vi "Write Image Header.vi"(8 "error in (no error)":errorcluster, 10 "Header Contents":T1={"FILENAME"=["FILENAME", "example.fits", "File name at acquisition"], "OBSERVER"=["OBSERVER", "Denis", "Observer’s (PI) name"], "PROGRID"=["PROGRID", "2018A-001", "Program ID"], "OBJECT"=["OBJECT", "UNDEFINED", "Object name"], "NIGHTDIR"=["NIGHTDIR", "DIR", "Night directory name "], "CHANNEL"=["CHANNEL", "RED", "Instrument channel"], "INSTRUME"=["INSTRUME", "ECHARPE", "Instrument"], "NEXPSEQ"=["NEXPSEQ", "1", "Total number of exposures in sequence"], "SEQINDEX"=["SEQINDEX", "1", "Exposure index in the sequence"], "OBSTYPE"=["OBSTYPE", "BIAS", "Image type: OBJECT, BIAS, FLAT, ARC, DARK"], "READMOD"=["READMOD", "Normal", "Read out mode: fast, normal, slow"], "SHUTTER"=["SHUTTER", "CLOSED", "Shutter Mode (OPEN, CLOSED, or AUTO) "], "OPENSHT"=["OPENSHT", "50", "Time to open the shutter (ms) "], "CLOSESHT"=["CLOSESHT", "50", "Time to close the shutter (ms)"], "GAIN"=["GAIN", "3.38", "Gain (e-/ADU)"], "GAINERR "=["GAINERR", "0.05", " Gain error (e-/ADU)"], "RDNOISE"=["RDNOISE", "6.55", "Read noise (e-)"], "RNOISERR"=["RNOISERR", "0.02", "Read noise error (e-)"], "SKYFIBER"=["SKYFIBER", "\"OFF\"", "Sky fiber: ON or OFF"], "CALFIBER"=["CALFIBER", "\"OFF\"", "Calibration Fiber: ON or OFF"], "UTDATE"=["UTDATE", "'2017-10-01T20", "UT date at start of exposure"], "LOCTIME"=["LOCTIME", "'2017-10-01T17", "LT date at start of exposure"], "MJD"=["MJD", "58027.500000", "Modified Julian Date at start of exposure"], "OBSLON"=["OBSLON", "-45.57972", "Observatory East Longitude"], "OBSLAT"=["OBSLAT", "-22.53444", "Observatory Latitude"], "OBSALT"=["OBSALT", "1864.0", "Observatory elevation above sea level (m)"], "EXPTIME"=["EXPTIME", "1", "Exposure time (s)"], "TELRA"=["TELRA", "“00:00:00.000”", "TCS right ascension: “HH:MM:SS.SSS”"], "TELDEC"=["TELDEC", "“+00:00:00.000”", "TCS declination: “+-DD:MM:SS.SSS”"], "RA"=["RA", "“00:00:00.000”", "Requested right Ascension: “HH:MM:SS.SSS”"], "DEC"=["DEC", "“+00:00:00.000”", "Requested Declination: “+- DD:MM:SS.SSS”"], "RA_DEG"=["RA_DEG", "128.84946", "Requested Right Ascension (deg)"], "DEC_DEG"=["DEC_DEG", "+19.648717", "Requested Declination (deg)"], "EPOCH"=["EPOCH", "2000.00", "Epoch for Target coordinates"], "HA"=["HA", "“+01:13:05.98”", "Hour Angle (Sexagesimal)"], "HAD"=["HAD", "1.2183292", "Hour Angle (deg)"], "AIRMASS"=["AIRMASS", "1.085", "Mean airmass for the observation"], "AMSTART"=["AMSTART", "1.060", "Airmass at start of exposure"], "AMEND"=["AMEND", "1.114", "Airmass at end of exposure"], "XOFFSET"=["XOFFSET", "0.000000", "Telescope RA offset in arcsec"], "YOFFSET"=["YOFFSET", "0.000000", "Telescope DEC offset in arcsec"], "PA"=["PA", "14.6415392418", "Current Rotator Position Angle (degree)"], "CAMFOC"=["CAMFOC", "-3.53", "Camera focus position (mm)"], "TELFOC"=["TELFOC", "-3.53", "Telescope focus position (mm)"], "TCSUT"=["TCSUT", "‘23:17:24.8’", "TCS Universal Time"], "MOONDIST"=["MOONDIST", "60.0", "Moon angular distance to object (deg)"], "MOONALT"=["MOONALT", "15.0", "Moon elevation above horizon (deg)"], "MONNPHAS"=["MOONPHAS", "30.0", "Moon phase (deg)"], "ADC"=["ADC", "\"ON\"", "Atmospheric Dispersion Corrector: ON or OFF"], "ADCSPPED"=["ADCSPPED", "5.0", "ADC motor speed (rpm)"], "CALMIRR"=["CALMIRR", "\"OUT\"", "Calibration mirror position: IN or OUT"], "GUIDING"=["GUIDING", "“ON”", "Guider status: ON or OFF"], "GUIDTEXP"=["GUIDTEXP", "1.0", "Guider exposure time (s)"], "GUIDFREQ"=["GUIDFREQ", "1.0", "Guiding frequency (Hz)"], "GUIDOBJX"=["GUIDOBJX", "102.5", "Guiding object x position (pixel)"], "GUIDOBJY"=["GUIDOBJY", "300.3", "Guiding object y position (pixel)"], "AVGYCORR"=["AVGYCORR", "2.3", "Average correction in RA (arcsec)"], "AVGXCORR"=["AVGXCORR", "1.3", "Average correction in DEC (arcsec)"], "GFOCUS"=["GFOCUS", "3.0", "Guider focus position (mm)"], "THARLAMP"=["THARLAMP", "“OFF”", "Thorium-Argon lamp state: ON or OFF"], "HALLAMP"=["HALLAMP", "“OFF”", "Halogen lamp state: ON or OFF"], "AGITATOR"=["AGITATOR", "“ON”", "Fiber agitator: ON or OFF"], "THARMIRR"=["THARMIRR", "“SPECTROGRAPH”", "Th-Ar mirror position: SPECTROGRAPH or TELESCOPE"], "DSTATUS"=["DSTATUS", "‘OPEN’", "Dome Status: OPEN or CLOSED"], "DTEMP"=["DTEMP", "10.0", "Dome temperature (deg C)"], "DHUM"=["DHUM", "82.0", "Dome humidity (per cent)"], "DLAMP"=["DLAMP", "“OFF”", "Dome lamp: ON or OFF"], "DFLAT"=["DFLAT", "“OFF”", "Dome flat lamp: ON or OFF"], "TEMPEXT"=["TEMPEXT", "10.0", "External temperature (deg C)"], "PRESSURE"=["PRESSURE", "742.00", "Pressure (mbar)"], "HUMIDITY"=["HUMIDITY", "92.00", "Humidity (per cent)"], "WINDDIR"=["WINDDIR", "15.0", "Wind direction: North-eastward (deg)"], "WSPEED"=["WSPEED", "30.2", "Wind Speed (km/h)"], "TCSST"=["TCSST", "‘23:12:32.5’", "TCS Sideral Time"], "DPOS"=["DPOS", "0.00000", "Dome position (deg)"]}, 11 "CCDCamera in":refnum<class "CCDCamera.lvclass">) -> (0 "error out":errorcluster, 3 "CCDCamera out":refnum<class "CCDCamera.lvclass">)   [LabVIEW 2018, in "CCDCamera.lvclass"]
doc: "This VI writes the provided information to the image header."
uses:
  CCDCamera.lvclass
  CCDCamera.lvclass/CCDCamera.ctl
  <userlib>/gfitsio/gfitsio-write-key-string.vi
  <userlib>/gfitsio/gfitsio.lvlib
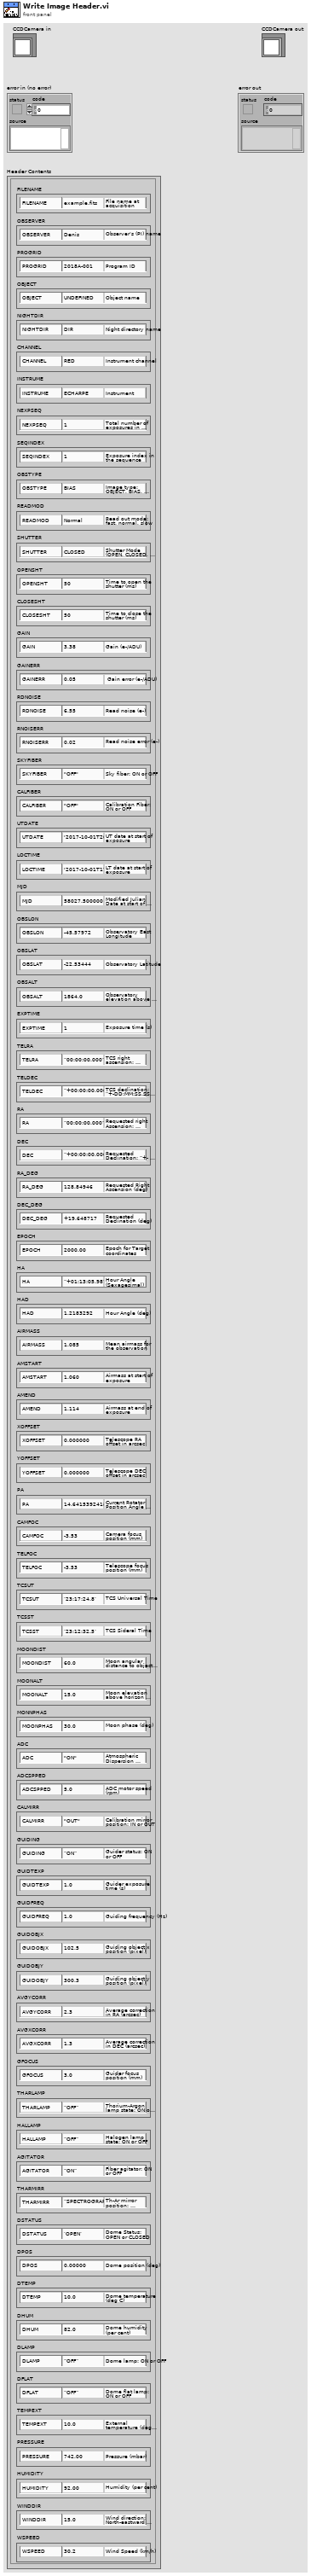
[diagram p1: front panel]
types:
  T1 = cluster{"FILENAME":string[], "OBSERVER":string[], "PROGRID":string[], "OBJECT":string[], "NIGHTDIR":string[], "CHANNEL":string[], "INSTRUME":string[], "NEXPSEQ":string[], "SEQINDEX":string[], "OBSTYPE":string[], "READMOD":string[], "SHUTTER":string[], "OPENSHT":string[], "CLOSESHT":string[], "GAIN":string[], "GAINERR ":string[], "RDNOISE":string[], "RNOISERR":string[], "SKYFIBER":string[], "CALFIBER":string[], "UTDATE":string[], "LOCTIME":string[], "MJD":string[], "OBSLON":string[], "OBSLAT":string[], "OBSALT":string[], "EXPTIME":string[], "TELRA":string[], "TELDEC":string[], "RA":string[], "DEC":string[], "RA_DEG":string[], "DEC_DEG":string[], "EPOCH":string[], "HA":string[], "HAD":string[], "AIRMASS":string[], "AMSTART":string[], "AMEND":string[], "XOFFSET":string[], "YOFFSET":string[], "PA":string[], "CAMFOC":string[], "TELFOC":string[], "TCSUT":string[], "MOONDIST":string[], "MOONALT":string[], "MONNPHAS":string[], "ADC":string[], "ADCSPPED":string[], "CALMIRR":string[], "GUIDING":string[], "GUIDTEXP":string[], "GUIDFREQ":string[], "GUIDOBJX":string[], "GUIDOBJY":string[], "AVGYCORR":string[], "AVGXCORR":string[], "GFOCUS":string[], "THARLAMP":string[], "HALLAMP":string[], "AGITATOR":string[], "THARMIRR":string[], "DSTATUS":string[], "DTEMP":string[], "DHUM":string[], "DLAMP":string[], "DFLAT":string[], "TEMPEXT":string[], "PRESSURE":string[], "HUMIDITY":string[], "WINDDIR":string[], "WSPEED":string[], "TCSST":string[], "DPOS":string[]}
  T2 = enum16{"open", "open or create", "create or replace", "create", "open (read only)"}
  T3 = typedef "gfitsio.lvlib/gfitsio-refnum.ctl" = refnum<k1>
diagram:
  (unwired) string[][] [["FILENAME", "example.fits", "File name at acquisition", "OBSTYPE", "UTDATE", "LOCTIME", "MJD", "OBSLON", "OBSLAT", "OBSALT", "NOME", "NOME", "NOME", "NOME", "NOME", "NOME", "NOME"], ["OBSERVER", "Denis", "Observer’s (PI) name", "NOME", "NOME", "NOME", "NOME", "NOME", "NOME", "NOME", "NOME", "NOME", "NOME", "NOME", "NOME", "NOME", "NOME"], ["PROGRID", "2018A-001", "Program ID", "NOME", "NOME", "NOME", "NOME", "NOME", "NOME", "NOME", "NOME", "NOME", "NOME", "NOME", "NOME", "NOME", "NOME"], ["OBJECT", "BIAS", "Object name", "NOME", "NOME", "NOME", "NOME", "NOME", "NOME", "NOME", "NOME", "NOME", "NOME", "NOME", "NOME", "NOME", "NOME"], ["NIGHTDIR ", "DIR ", "Night directory name ", "", "", "", "", "", "", "", "", "", "", "", "", "", ""], ["CHANNEL", "RED", "Instrument channel", "NOME", "NOME", "NOME", "NOME", "NOME", "NOME", "NOME", "NOME", "NOME", "NOME", "NOME", "NOME", "NOME", "NOME"], ["INSTRUME", "SPARC4", "Instrument", "NOME", "NOME", "NOME", "NOME", "NOME", "NOME", "NOME", "NOME", "NOME", "NOME", "NOME", "NOME", "NOME", "NOME"], ["NEXPSEQ", "NONE", "Total number of exposures in sequence", "NOME", "NOME", "NOME", "NOME", "NOME", "NOME", "NOME", "NOME", "NOME", "NOME", "NOME", "NOME", "NOME", "NOME"], ["SEQINDEX", "NONE", "Exposure index in the sequence", "NOME", "NOME", "NOME", "NOME", "NOME", "NOME", "NOME", "NOME", "NOME", "NOME", "NOME", "NOME", "NOME", "NOME"], ["OBSTYPE", "Bias", "Image type: OBJECT, BIAS, FLAT, ARC, DARK", "NOME", "NOME", "NOME", "NOME", "NOME", "NOME", "NOME", "NOME", "NOME", "NOME", "NOME", "NOME", "NOME", "NOME"], ["READMOD", "Normal", "Read out mode: fast, normal, slow", "NOME", "NOME", "NOME", "NOME", "NOME", "NOME", "NOME", "NOME", "NOME", "NOME", "NOME", "NOME", "NOME", "NOME"], ["SHUTTER ", " ", "Shutter Mode (OPEN, CLOSED, or AUTO) ", "", "", "", "", "", "", "", "", "", "", "", "", "", ""], ["OPENSHT ", " ", "Time to open the shutter (ms) ", "", "", "", "", "", "", "", "", "", "", "", "", "", ""], ["CLOSESHT", "", "Time to close the shutter (ms)", "NOME", "NOME", "NOME", "NOME", "NOME", "NOME", "NOME", "NOME", "NOME", "NOME", "NOME", "NOME", "NOME", "NOME"], ["GAIN", "3.38", "Gain (e-/ADU)", "NOME", "NOME", "NOME", "NOME", "NOME", "NOME", "NOME", "NOME", "NOME", "NOME", "NOME", "NOME", "NOME", "NOME"], ["GAINERR ", "0.05 ", " Gain error (e-/ADU)", "", "", "", "", "", "", "", "", "", "", "", "", "", ""], ["RDNOISE", "6.55", "Read noise (e-)", "NOME", "NOME", "NOME", "NOME", "NOME", "NOME", "NOME", "NOME", "NOME", "NOME", "NOME", "NOME", "NOME", "NOME"], ["RNOISERR", "0.02", "Read noise error (e-)", "NOME", "NOME", "NOME", "NOME", "NOME", "NOME", "NOME", "NOME", "NOME", "NOME", "NOME", "NOME", "NOME", "NOME"], ["SKYFIBER", "OFF", "Sky fiber: ON or OFF", "NOME", "NOME", "NOME", "NOME", "NOME", "NOME", "NOME", "NOME", "NOME", "NOME", "NOME", "NOME", "NOME", "NOME"], ["CALFIBER", "OFF", "Calibration Fiber: ON or OFF", "NOME", "NOME", "NOME", "NOME", "NOME", "NOME", "NOME", "NOME", "NOME", "NOME", "NOME", "NOME", "NOME", "NOME"], ["UTDATE", "'2017-10-01T20:34:3 6.000'", "UT date at start of exposure", "NOME", "NOME", "NOME", "NOME", "NOME", "NOME", "NOME", "NOME", "NOME", "NOME", "NOME", "NOME", "NOME", "NOME"], ["LOCTIME", "'2017-10-01T17:34:3 6.000'", "LT date at start of exposure", "NOME", "NOME", "NOME", "NOME", "NOME", "NOME", "NOME", "NOME", "NOME", "NOME", "NOME", "NOME", "NOME", "NOME"], ["MJD", "58027.500000", "Modified Julian Date at start of exposure", "NOME", "NOME", "NOME", "NOME", "NOME", "NOME", "NOME", "NOME", "NOME", "NOME", "NOME", "NOME", "NOME", "NOME"], ["OBSLON", "-45.57972", "Observatory East Longitude", "NOME", "NOME", "NOME", "NOME", "NOME", "NOME", "NOME", "NOME", "NOME", "NOME", "NOME", "NOME", "NOME", "NOME"], ["OBSLAT", "-22.53444", "Observatory Latitude", "NOME", "NOME", "NOME", "NOME", "NOME", "NOME", "NOME", "NOME", "NOME", "NOME", "NOME", "NOME", "NOME", "NOME"], ["OBSALT", "1864.0", "Observatory elevation above sea level (m)", "NOME", "NOME", "NOME", "NOME", "NOME", "NOME", "NOME", "NOME", "NOME", "NOME", "NOME", "NOME", "NOME", "NOME"], ["EXPTIME", "0.0", "Exposure time (s)", "NOME", "NOME", "NOME", "NOME", "NOME", "NOME", "NOME", "NOME", "NOME", "NOME", "NOME", "NOME", "NOME", "NOME"], ["TELRA", "“00:00:00.000”", "TCS right ascension: “HH:MM:SS.SSS”", "NOME", "NOME", "NOME", "NOME", "NOME", "NOME", "NOME", "NOME", "NOME", "NOME", "NOME", "NOME", "NOME", "NOME"], ["TELDEC", "“+00:00:00.000”", "TCS declination: “+-DD:MM:SS.SSS”", "NOME", "NOME", "NOME", "NOME", "NOME", "NOME", "NOME", "NOME", "NOME", "NOME", "NOME", "NOME", "NOME", "NOME"], ["RA", "“00:00:00.000”", "Requested right Ascension: “HH:MM:SS.SSS”", "NOME", "NOME", "NOME", "NOME", "NOME", "NOME", "NOME", "NOME", "NOME", "NOME", "NOME", "NOME", "NOME", "NOME"], ["DEC", "“+00:00:00.000”", "Requested Declination: “+- DD:MM:SS.SSS”", "NOME", "NOME", "NOME", "NOME", "NOME", "NOME", "NOME", "NOME", "NOME", "NOME", "NOME", "NOME", "NOME", "NOME"], ["RA_DEG", "128.84946", "Requested Right Ascension (deg)", "NOME", "NOME", "NOME", "NOME", "NOME", "NOME", "NOME", "NOME", "NOME", "NOME", "NOME", "NOME", "NOME", "NOME"], ["DEC_DEG", "+19.648717", "Requested Declination (deg)", "NOME", "NOME", "NOME", "NOME", "NOME", "NOME", "NOME", "NOME", "NOME", "NOME", "NOME", "NOME", "NOME", "NOME"], ["EPOCH", "2000.00", "Epoch for Target coordinates", "NOME", "NOME", "NOME", "NOME", "NOME", "NOME", "NOME", "NOME", "NOME", "NOME", "NOME", "NOME", "NOME", "NOME"], ["HA", "“+01:13:05.98”", "Hour Angle (Sexagesimal)", "NOME", "NOME", "NOME", "NOME", "NOME", "NOME", "NOME", "NOME", "NOME", "NOME", "NOME", "NOME", "NOME", "NOME"], ["HAD", "1.2183292", "Hour Angle (deg)", "NOME", "NOME", "NOME", "NOME", "NOME", "NOME", "NOME", "NOME", "NOME", "NOME", "NOME", "NOME", "NOME", "NOME"], ["AIRMASS", "1.085", "Mean airmass for the observation", "NOME", "NOME", "NOME", "NOME", "NOME", "NOME", "NOME", "NOME", "NOME", "NOME", "NOME", "NOME", "NOME", "NOME"], ["AMSTART", "1.060", "Airmass at start of exposure", "NOME", "NOME", "NOME", "NOME", "NOME", "NOME", "NOME", "NOME", "NOME", "NOME", "NOME", "NOME", "NOME", "NOME"], ["AMEND", "1.114", "Airmass at end of exposure", "NOME", "NOME", "NOME", "NOME", "NOME", "NOME", "NOME", "NOME", "NOME", "NOME", "NOME", "NOME", "NOME", "NOME"], ["XOFFSET", "0.000000", "Telescope RA offset in arcsec", "NOME", "NOME", "NOME", "NOME", "NOME", "NOME", "NOME", "NOME", "NOME", "NOME", "NOME", "NOME", "NOME", "NOME"], ["YOFFSET", "0.000000", "Telescope DEC offset in arcsec", "NOME", "NOME", "NOME", "NOME", "NOME", "NOME", "NOME", "NOME", "NOME", "NOME", "NOME", "NOME", "NOME", "NOME"], ["PA", "14.6415392418", "Current Rotator Position Angle (degree)", "NOME", "NOME", "NOME", "NOME", "NOME", "NOME", "NOME", "NOME", "NOME", "NOME", "NOME", "NOME", "NOME", "NOME"], ["CAMFOC", "-3.53", "Camera focus position (mm)", "NOME", "NOME", "NOME", "NOME", "NOME", "NOME", "NOME", "NOME", "NOME", "NOME", "NOME", "NOME", "NOME", "NOME"], ["TELFOC", "-3.53", "Telescope focus position (mm)", "NOME", "NOME", "NOME", "NOME", "NOME", "NOME", "NOME", "NOME", "NOME", "NOME", "NOME", "NOME", "NOME", "NOME"], ["TCSUT", "‘23:17:24.8’", "TCS Universal Time", "NOME", "NOME", "NOME", "NOME", "NOME", "NOME", "NOME", "NOME", "NOME", "NOME", "NOME", "NOME", "NOME", "NOME"], ["TCSST", "‘23:12:32.5’", "TCS Sideral Time", "NOME", "NOME", "NOME", "NOME", "NOME", "NOME", "NOME", "NOME", "NOME", "NOME", "NOME", "NOME", "NOME", "NOME"], ["MOONDIST", "60.0", "Moon angular distance to object (deg)", "NOME", "NOME", "NOME", "NOME", "NOME", "NOME", "NOME", "NOME", "NOME", "NOME", "NOME", "NOME", "NOME", "NOME"], ["MOONALT", "15.0", "Moon elevation above horizon (deg)", "NOME", "NOME", "NOME", "NOME", "NOME", "NOME", "NOME", "NOME", "NOME", "NOME", "NOME", "NOME", "NOME", "NOME"], ["MOONPHAS", "30.0", "Moon phase (deg)", "NOME", "NOME", "NOME", "NOME", "NOME", "NOME", "NOME", "NOME", "NOME", "NOME", "NOME", "NOME", "NOME", "NOME"], ["ADC", "\"ON\"", "Atmospheric Dispersion Corrector: ON or OFF", "NOME", "NOME", "NOME", "NOME", "NOME", "NOME", "NOME", "NOME", "NOME", "NOME", "NOME", "NOME", "NOME", "NOME"], ["ADCSPPED", "5.0", "ADC motor speed (rpm)", "NOME", "NOME", "NOME", "NOME", "NOME", "NOME", "NOME", "NOME", "NOME", "NOME", "NOME", "NOME", "NOME", "NOME"], ["CALMIRR", "\"OUT\"", "Calibration mirror position: IN or OUT", "NOME", "NOME", "NOME", "NOME", "NOME", "NOME", "NOME", "NOME", "NOME", "NOME", "NOME", "NOME", "NOME", "NOME"], ["GUIDING", "“ON”", "Guider status: ON or OFF", "NOME", "NOME", "NOME", "NOME", "NOME", "NOME", "NOME", "NOME", "NOME", "NOME", "NOME", "NOME", "NOME", "NOME"], ["GUIDTEXP", "1.0", "Guider exposure time (s)", "NOME", "NOME", "NOME", "NOME", "NOME", "NOME", "NOME", "NOME", "NOME", "NOME", "NOME", "NOME", "NOME", "NOME"], ["GUIDFREQ", "1.0", "Guiding frequency (Hz)", "NOME", "NOME", "NOME", "NOME", "NOME", "NOME", "NOME", "NOME", "NOME", "NOME", "NOME", "NOME", "NOME", "NOME"], ["GUIDOBJX", "102.5", "Guiding object x position (pixel)", "NOME", "NOME", "NOME", "NOME", "NOME", "NOME", "NOME", "NOME", "NOME", "NOME", "NOME", "NOME", "NOME", "NOME"], ["GUIDOBJY", "300.3", "Guiding object y position (pixel)", "NOME", "NOME", "NOME", "NOME", "NOME", "NOME", "NOME", "NOME", "NOME", "NOME", "NOME", "NOME", "NOME", "NOME"], ["AVGYCORR", "2.3", "Average correction in RA (arcsec)", "NOME", "NOME", "NOME", "NOME", "NOME", "NOME", "NOME", "NOME", "NOME", "NOME", "NOME", "NOME", "NOME", "NOME"], ["AVGXCORR", "1.3", "Average correction in DEC (arcsec)", "NOME", "NOME", "NOME", "NOME", "NOME", "NOME", "NOME", "NOME", "NOME", "NOME", "NOME", "NOME", "NOME", "NOME"], ["GFOCUS", "3.0", "Guider focus position (mm)", "NOME", "NOME", "NOME", "NOME", "NOME", "NOME", "NOME", "NOME", "NOME", "NOME", "NOME", "NOME", "NOME", "NOME"], ["THARLAMP", "“OFF”", "Thorium-Argon lamp state: ON or OFF", "NOME", "NOME", "NOME", "NOME", "NOME", "NOME", "NOME", "NOME", "NOME", "NOME", "NOME", "NOME", "NOME", "NOME"], ["HALLAMP", "“OFF”", "Halogen lamp state: ON or OFF", "NOME", "NOME", "NOME", "NOME", "NOME", "NOME", "NOME", "NOME", "NOME", "NOME", "NOME", "NOME", "NOME", "NOME"], ["AGITATOR", "“ON”", "Fiber agitator: ON or OFF", "NOME", "NOME", "NOME", "NOME", "NOME", "NOME", "NOME", "NOME", "NOME", "NOME", "NOME", "NOME", "NOME", "NOME"], ["THARMIRR", "“SPECTROGRAPH”", "Th-Ar mirror position: SPECTROGRAPH or TELESCOPE", "NOME", "NOME", "NOME", "NOME", "NOME", "NOME", "NOME", "NOME", "NOME", "NOME", "NOME", "NOME", "NOME", "NOME"], ["DSTATUS", "‘OPEN’", "Dome Status: OPEN or CLOSED", "NOME", "NOME", "NOME", "NOME", "NOME", "NOME", "NOME", "NOME", "NOME", "NOME", "NOME", "NOME", "NOME", "NOME"], ["DPOS", "0.00000", "Dome position (deg)", "NOME", "NOME", "NOME", "NOME", "NOME", "NOME", "NOME", "NOME", "NOME", "NOME", "NOME", "NOME", "NOME", "NOME"], ["DTEMP", "10.0", "Dome temperature (deg C)", "NOME", "NOME", "NOME", "NOME", "NOME", "NOME", "NOME", "NOME", "NOME", "NOME", "NOME", "NOME", "NOME", "NOME"], ["DHUM", "82.0", "Dome humidity (per cent)", "NOME", "NOME", "NOME", "NOME", "NOME", "NOME", "NOME", "NOME", "NOME", "NOME", "NOME", "NOME", "NOME", "NOME"], ["DLAMP", "“OFF”", "Dome lamp: ON or OFF", "NOME", "NOME", "NOME", "NOME", "NOME", "NOME", "NOME", "NOME", "NOME", "NOME", "NOME", "NOME", "NOME", "NOME"], ["DFLAT", "“OFF”", "Dome flat lamp: ON or OFF", "NOME", "NOME", "NOME", "NOME", "NOME", "NOME", "NOME", "NOME", "NOME", "NOME", "NOME", "NOME", "NOME", "NOME"], ["TEMPEXT", "10.0", "External temperature (deg C)", "NOME", "NOME", "NOME", "NOME", "NOME", "NOME", "NOME", "NOME", "NOME", "NOME", "NOME", "NOME", "NOME", "NOME"], ["PRESSURE", "742.00", "Pressure (mbar)", "NOME", "NOME", "NOME", "NOME", "NOME", "NOME", "NOME", "NOME", "NOME", "NOME", "NOME", "NOME", "NOME", "NOME"], ["HUMIDITY", "92.00", "Humidity (per cent)", "NOME", "NOME", "NOME", "NOME", "NOME", "NOME", "NOME", "NOME", "NOME", "NOME", "NOME", "NOME", "NOME", "NOME"], ["WINDDIR", "15.0", "Wind direction: North-eastward (deg)", "NOME", "NOME", "NOME", "NOME", "NOME", "NOME", "NOME", "NOME", "NOME", "NOME", "NOME", "NOME", "NOME", "NOME"], ["WSPEED", "30.2", "Wind Speed (km/h)", "NOME", "NOME", "NOME", "NOME", "NOME", "NOME", "NOME", "NOME", "NOME", "NOME", "NOME", "NOME", "NOME", "NOME"]] ("Table of the header")
  (unwired) string[][] [["FILENAME", "example.fits", "File name at acquisition", "OBSTYPE", "UTDATE", "LOCTIME", "MJD", "OBSLON", "OBSLAT", "OBSALT", "NOME", "NOME", "NOME", "NOME", "NOME", "NOME", "NOME"], ["OBSERVER", "Denis", "Observer’s (PI) name", "NOME", "NOME", "NOME", "NOME", "NOME", "NOME", "NOME", "NOME", "NOME", "NOME", "NOME", "NOME", "NOME", "NOME"], ["PROGRID", "2018A-001", "Program ID", "NOME", "NOME", "NOME", "NOME", "NOME", "NOME", "NOME", "NOME", "NOME", "NOME", "NOME", "NOME", "NOME", "NOME"], ["OBJECT", "BIAS", "Object name", "NOME", "NOME", "NOME", "NOME", "NOME", "NOME", "NOME", "NOME", "NOME", "NOME", "NOME", "NOME", "NOME", "NOME"], ["NIGHTDIR ", "DIR ", "Night directory name ", "", "", "", "", "", "", "", "", "", "", "", "", "", ""], ["CHANNEL", "RED", "Instrument channel", "NOME", "NOME", "NOME", "NOME", "NOME", "NOME", "NOME", "NOME", "NOME", "NOME", "NOME", "NOME", "NOME", "NOME"], ["INSTRUME", "SPARC4", "Instrument", "NOME", "NOME", "NOME", "NOME", "NOME", "NOME", "NOME", "NOME", "NOME", "NOME", "NOME", "NOME", "NOME", "NOME"], ["NEXPSEQ", "NONE", "Total number of exposures in sequence", "NOME", "NOME", "NOME", "NOME", "NOME", "NOME", "NOME", "NOME", "NOME", "NOME", "NOME", "NOME", "NOME", "NOME"], ["SEQINDEX", "NONE", "Exposure index in the sequence", "NOME", "NOME", "NOME", "NOME", "NOME", "NOME", "NOME", "NOME", "NOME", "NOME", "NOME", "NOME", "NOME", "NOME"], ["OBSTYPE", "Bias", "Image type: OBJECT, BIAS, FLAT, ARC, DARK", "NOME", "NOME", "NOME", "NOME", "NOME", "NOME", "NOME", "NOME", "NOME", "NOME", "NOME", "NOME", "NOME", "NOME"], ["READMOD", "Normal", "Read out mode: fast, normal, slow", "NOME", "NOME", "NOME", "NOME", "NOME", "NOME", "NOME", "NOME", "NOME", "NOME", "NOME", "NOME", "NOME", "NOME"], ["SHUTTER ", " ", "Shutter Mode (OPEN, CLOSED, or AUTO) ", "", "", "", "", "", "", "", "", "", "", "", "", "", ""], ["OPENSHT ", " ", "Time to open the shutter (ms) ", "", "", "", "", "", "", "", "", "", "", "", "", "", ""], ["CLOSESHT", "", "Time to close the shutter (ms)", "NOME", "NOME", "NOME", "NOME", "NOME", "NOME", "NOME", "NOME", "NOME", "NOME", "NOME", "NOME", "NOME", "NOME"], ["GAIN", "3.38", "Gain (e-/ADU)", "NOME", "NOME", "NOME", "NOME", "NOME", "NOME", "NOME", "NOME", "NOME", "NOME", "NOME", "NOME", "NOME", "NOME"], ["GAINERR ", "0.05 ", " Gain error (e-/ADU)", "", "", "", "", "", "", "", "", "", "", "", "", "", ""], ["RDNOISE", "6.55", "Read noise (e-)", "NOME", "NOME", "NOME", "NOME", "NOME", "NOME", "NOME", "NOME", "NOME", "NOME", "NOME", "NOME", "NOME", "NOME"], ["RNOISERR", "0.02", "Read noise error (e-)", "NOME", "NOME", "NOME", "NOME", "NOME", "NOME", "NOME", "NOME", "NOME", "NOME", "NOME", "NOME", "NOME", "NOME"], ["SKYFIBER", "OFF", "Sky fiber: ON or OFF", "NOME", "NOME", "NOME", "NOME", "NOME", "NOME", "NOME", "NOME", "NOME", "NOME", "NOME", "NOME", "NOME", "NOME"], ["CALFIBER", "OFF", "Calibration Fiber: ON or OFF", "NOME", "NOME", "NOME", "NOME", "NOME", "NOME", "NOME", "NOME", "NOME", "NOME", "NOME", "NOME", "NOME", "NOME"], ["UTDATE", "'2017-10-01T20:34:3 6.000'", "UT date at start of exposure", "NOME", "NOME", "NOME", "NOME", "NOME", "NOME", "NOME", "NOME", "NOME", "NOME", "NOME", "NOME", "NOME", "NOME"], ["LOCTIME", "'2017-10-01T17:34:3 6.000'", "LT date at start of exposure", "NOME", "NOME", "NOME", "NOME", "NOME", "NOME", "NOME", "NOME", "NOME", "NOME", "NOME", "NOME", "NOME", "NOME"], ["MJD", "58027.500000", "Modified Julian Date at start of exposure", "NOME", "NOME", "NOME", "NOME", "NOME", "NOME", "NOME", "NOME", "NOME", "NOME", "NOME", "NOME", "NOME", "NOME"], ["OBSLON", "-45.57972", "Observatory East Longitude", "NOME", "NOME", "NOME", "NOME", "NOME", "NOME", "NOME", "NOME", "NOME", "NOME", "NOME", "NOME", "NOME", "NOME"], ["OBSLAT", "-22.53444", "Observatory Latitude", "NOME", "NOME", "NOME", "NOME", "NOME", "NOME", "NOME", "NOME", "NOME", "NOME", "NOME", "NOME", "NOME", "NOME"], ["OBSALT", "1864.0", "Observatory elevation above sea level (m)", "NOME", "NOME", "NOME", "NOME", "NOME", "NOME", "NOME", "NOME", "NOME", "NOME", "NOME", "NOME", "NOME", "NOME"], ["EXPTIME", "0.0", "Exposure time (s)", "NOME", "NOME", "NOME", "NOME", "NOME", "NOME", "NOME", "NOME", "NOME", "NOME", "NOME", "NOME", "NOME", "NOME"], ["TELRA", "“00:00:00.000”", "TCS right ascension: “HH:MM:SS.SSS”", "NOME", "NOME", "NOME", "NOME", "NOME", "NOME", "NOME", "NOME", "NOME", "NOME", "NOME", "NOME", "NOME", "NOME"], ["TELDEC", "“+00:00:00.000”", "TCS declination: “+-DD:MM:SS.SSS”", "NOME", "NOME", "NOME", "NOME", "NOME", "NOME", "NOME", "NOME", "NOME", "NOME", "NOME", "NOME", "NOME", "NOME"], ["RA", "“00:00:00.000”", "Requested right Ascension: “HH:MM:SS.SSS”", "NOME", "NOME", "NOME", "NOME", "NOME", "NOME", "NOME", "NOME", "NOME", "NOME", "NOME", "NOME", "NOME", "NOME"], ["DEC", "“+00:00:00.000”", "Requested Declination: “+- DD:MM:SS.SSS”", "NOME", "NOME", "NOME", "NOME", "NOME", "NOME", "NOME", "NOME", "NOME", "NOME", "NOME", "NOME", "NOME", "NOME"], ["RA_DEG", "128.84946", "Requested Right Ascension (deg)", "NOME", "NOME", "NOME", "NOME", "NOME", "NOME", "NOME", "NOME", "NOME", "NOME", "NOME", "NOME", "NOME", "NOME"], ["DEC_DEG", "+19.648717", "Requested Declination (deg)", "NOME", "NOME", "NOME", "NOME", "NOME", "NOME", "NOME", "NOME", "NOME", "NOME", "NOME", "NOME", "NOME", "NOME"], ["EPOCH", "2000.00", "Epoch for Target coordinates", "NOME", "NOME", "NOME", "NOME", "NOME", "NOME", "NOME", "NOME", "NOME", "NOME", "NOME", "NOME", "NOME", "NOME"], ["HA", "“+01:13:05.98”", "Hour Angle (Sexagesimal)", "NOME", "NOME", "NOME", "NOME", "NOME", "NOME", "NOME", "NOME", "NOME", "NOME", "NOME", "NOME", "NOME", "NOME"], ["HAD", "1.2183292", "Hour Angle (deg)", "NOME", "NOME", "NOME", "NOME", "NOME", "NOME", "NOME", "NOME", "NOME", "NOME", "NOME", "NOME", "NOME", "NOME"], ["AIRMASS", "1.085", "Mean airmass for the observation", "NOME", "NOME", "NOME", "NOME", "NOME", "NOME", "NOME", "NOME", "NOME", "NOME", "NOME", "NOME", "NOME", "NOME"], ["AMSTART", "1.060", "Airmass at start of exposure", "NOME", "NOME", "NOME", "NOME", "NOME", "NOME", "NOME", "NOME", "NOME", "NOME", "NOME", "NOME", "NOME", "NOME"], ["AMEND", "1.114", "Airmass at end of exposure", "NOME", "NOME", "NOME", "NOME", "NOME", "NOME", "NOME", "NOME", "NOME", "NOME", "NOME", "NOME", "NOME", "NOME"], ["XOFFSET", "0.000000", "Telescope RA offset in arcsec", "NOME", "NOME", "NOME", "NOME", "NOME", "NOME", "NOME", "NOME", "NOME", "NOME", "NOME", "NOME", "NOME", "NOME"], ["YOFFSET", "0.000000", "Telescope DEC offset in arcsec", "NOME", "NOME", "NOME", "NOME", "NOME", "NOME", "NOME", "NOME", "NOME", "NOME", "NOME", "NOME", "NOME", "NOME"], ["PA", "14.6415392418", "Current Rotator Position Angle (degree)", "NOME", "NOME", "NOME", "NOME", "NOME", "NOME", "NOME", "NOME", "NOME", "NOME", "NOME", "NOME", "NOME", "NOME"], ["CAMFOC", "-3.53", "Camera focus position (mm)", "NOME", "NOME", "NOME", "NOME", "NOME", "NOME", "NOME", "NOME", "NOME", "NOME", "NOME", "NOME", "NOME", "NOME"], ["TELFOC", "-3.53", "Telescope focus position (mm)", "NOME", "NOME", "NOME", "NOME", "NOME", "NOME", "NOME", "NOME", "NOME", "NOME", "NOME", "NOME", "NOME", "NOME"], ["TCSUT", "‘23:17:24.8’", "TCS Universal Time", "NOME", "NOME", "NOME", "NOME", "NOME", "NOME", "NOME", "NOME", "NOME", "NOME", "NOME", "NOME", "NOME", "NOME"], ["TCSST", "‘23:12:32.5’", "TCS Sideral Time", "NOME", "NOME", "NOME", "NOME", "NOME", "NOME", "NOME", "NOME", "NOME", "NOME", "NOME", "NOME", "NOME", "NOME"], ["MOONDIST", "60.0", "Moon angular distance to object (deg)", "NOME", "NOME", "NOME", "NOME", "NOME", "NOME", "NOME", "NOME", "NOME", "NOME", "NOME", "NOME", "NOME", "NOME"], ["MOONALT", "15.0", "Moon elevation above horizon (deg)", "NOME", "NOME", "NOME", "NOME", "NOME", "NOME", "NOME", "NOME", "NOME", "NOME", "NOME", "NOME", "NOME", "NOME"], ["MONNPHAS", "30.0", "Moon phase (deg)", "NOME", "NOME", "NOME", "NOME", "NOME", "NOME", "NOME", "NOME", "NOME", "NOME", "NOME", "NOME", "NOME", "NOME"], ["ADC", "\"ON\"", "Atmospheric Dispersion Corrector: ON or OFF", "NOME", "NOME", "NOME", "NOME", "NOME", "NOME", "NOME", "NOME", "NOME", "NOME", "NOME", "NOME", "NOME", "NOME"], ["ADCSPPED", "5.0", "ADC motor speed (rpm)", "NOME", "NOME", "NOME", "NOME", "NOME", "NOME", "NOME", "NOME", "NOME", "NOME", "NOME", "NOME", "NOME", "NOME"], ["CALMIRR", "\"OUT\"", "Calibration mirror position: IN or OUT", "NOME", "NOME", "NOME", "NOME", "NOME", "NOME", "NOME", "NOME", "NOME", "NOME", "NOME", "NOME", "NOME", "NOME"], ["GUIDING", "“ON”", "Guider status: ON or OFF", "NOME", "NOME", "NOME", "NOME", "NOME", "NOME", "NOME", "NOME", "NOME", "NOME", "NOME", "NOME", "NOME", "NOME"], ["GUIDTEXP", "1.0", "Guider exposure time (s)", "NOME", "NOME", "NOME", "NOME", "NOME", "NOME", "NOME", "NOME", "NOME", "NOME", "NOME", "NOME", "NOME", "NOME"], ["GUIDFREQ", "1.0", "Guiding frequency (Hz)", "NOME", "NOME", "NOME", "NOME", "NOME", "NOME", "NOME", "NOME", "NOME", "NOME", "NOME", "NOME", "NOME", "NOME"], ["GUIDOBJX", "102.5", "Guiding object x position (pixel)", "NOME", "NOME", "NOME", "NOME", "NOME", "NOME", "NOME", "NOME", "NOME", "NOME", "NOME", "NOME", "NOME", "NOME"], ["GUIDOBJY", "300.3", "Guiding object y position (pixel)", "NOME", "NOME", "NOME", "NOME", "NOME", "NOME", "NOME", "NOME", "NOME", "NOME", "NOME", "NOME", "NOME", "NOME"], ["AVGYCORR", "2.3", "Average correction in RA (arcsec)", "NOME", "NOME", "NOME", "NOME", "NOME", "NOME", "NOME", "NOME", "NOME", "NOME", "NOME", "NOME", "NOME", "NOME"], ["AVGXCORR", "1.3", "Average correction in DEC (arcsec)", "NOME", "NOME", "NOME", "NOME", "NOME", "NOME", "NOME", "NOME", "NOME", "NOME", "NOME", "NOME", "NOME", "NOME"], ["GFOCUS", "3.0", "Guider focus position (mm)", "NOME", "NOME", "NOME", "NOME", "NOME", "NOME", "NOME", "NOME", "NOME", "NOME", "NOME", "NOME", "NOME", "NOME"], ["THARLAMP", "“OFF”", "Thorium-Argon lamp state: ON or OFF", "NOME", "NOME", "NOME", "NOME", "NOME", "NOME", "NOME", "NOME", "NOME", "NOME", "NOME", "NOME", "NOME", "NOME"], ["HALLAMP", "“OFF”", "Halogen lamp state: ON or OFF", "NOME", "NOME", "NOME", "NOME", "NOME", "NOME", "NOME", "NOME", "NOME", "NOME", "NOME", "NOME", "NOME", "NOME"], ["AGITATOR", "“ON”", "Fiber agitator: ON or OFF", "NOME", "NOME", "NOME", "NOME", "NOME", "NOME", "NOME", "NOME", "NOME", "NOME", "NOME", "NOME", "NOME", "NOME"], ["THARMIRR", "“SPECTROGRAPH”", "Th-Ar mirror position: SPECTROGRAPH or TELESCOPE", "NOME", "NOME", "NOME", "NOME", "NOME", "NOME", "NOME", "NOME", "NOME", "NOME", "NOME", "NOME", "NOME", "NOME"], ["DSTATUS", "‘OPEN’", "Dome Status: OPEN or CLOSED", "NOME", "NOME", "NOME", "NOME", "NOME", "NOME", "NOME", "NOME", "NOME", "NOME", "NOME", "NOME", "NOME", "NOME"], ["DPOS", "0.00000", "Dome position (deg)", "NOME", "NOME", "NOME", "NOME", "NOME", "NOME", "NOME", "NOME", "NOME", "NOME", "NOME", "NOME", "NOME", "NOME"], ["DTEMP", "10.0", "Dome temperature (deg C)", "NOME", "NOME", "NOME", "NOME", "NOME", "NOME", "NOME", "NOME", "NOME", "NOME", "NOME", "NOME", "NOME", "NOME"], ["DHUM", "82.0", "Dome humidity (per cent)", "NOME", "NOME", "NOME", "NOME", "NOME", "NOME", "NOME", "NOME", "NOME", "NOME", "NOME", "NOME", "NOME", "NOME"], ["DLAMP", "“OFF”", "Dome lamp: ON or OFF", "NOME", "NOME", "NOME", "NOME", "NOME", "NOME", "NOME", "NOME", "NOME", "NOME", "NOME", "NOME", "NOME", "NOME"], ["DFLAT", "“OFF”", "Dome flat lamp: ON or OFF", "NOME", "NOME", "NOME", "NOME", "NOME", "NOME", "NOME", "NOME", "NOME", "NOME", "NOME", "NOME", "NOME", "NOME"], ["TEMPEXT", "10.0", "External temperature (deg C)", "NOME", "NOME", "NOME", "NOME", "NOME", "NOME", "NOME", "NOME", "NOME", "NOME", "NOME", "NOME", "NOME", "NOME"], ["PRESSURE", "742.00", "Pressure (mbar)", "NOME", "NOME", "NOME", "NOME", "NOME", "NOME", "NOME", "NOME", "NOME", "NOME", "NOME", "NOME", "NOME", "NOME"], ["HUMIDITY", "92.00", "Humidity (per cent)", "NOME", "NOME", "NOME", "NOME", "NOME", "NOME", "NOME", "NOME", "NOME", "NOME", "NOME", "NOME", "NOME", "NOME"], ["WINDDIR", "15.0", "Wind direction: North-eastward (deg)", "NOME", "NOME", "NOME", "NOME", "NOME", "NOME", "NOME", "NOME", "NOME", "NOME", "NOME", "NOME", "NOME", "NOME"], ["WSPEED", "30.2", "Wind Speed (km/h)", "NOME", "NOME", "NOME", "NOME", "NOME", "NOME", "NOME", "NOME", "NOME", "NOME", "NOME", "NOME", "NOME", "NOME"]] ("Table of the header")
  (unwired) i32[] [1, 2, 3, 4, 5, 6, 7, 8, 9, 10, 11, 12, 13, 14, 15, 16, 17, 18, 19, 20, 21, 22, 23, 24, 25, 26, 27, 28, 29, 30, 31, 32, 33, 34, 35, 36, 37, 38, 39, 40, 41, 42, 43, 44, 45, 46, 47, 48, 49, 50, 51, 52, 53, 54, 55, 56, 57, 58, 59, 60, 61, 62, 63, 64, 65, 66, 67, 68, 69, 70, 71]
  n1 = stacked-sequence {
    tunnel: "CCDCamera in" -> [w6]
    tunnel: [w6] -> w1
    frame #0 {
      n2 = Unbundle By Name(w6) -> ("Last Image"=w10:string)
      n3 = Unbundle By Name("Header Contents") -> ("FILENAME"=w8:string[])
      n4 = local read "Header Contents"() -> (w12:T1)
      n5 = Replace Array Subset(array=w8, new element=w10, index=1) -> (w13:string[])
      n6 = Bundle By Name(cluster=w12, "FILENAME"=w13) -> (w11:T1)
      n7 = local write "Header Contents"(w11) -> ()
    }
  }
  n8 = case shown="No Error" "error in (no error)" {
    selector: "error in (no error)" -> [w701 w703]
    tunnel: [w699 w703] -> w4
    tunnel: [w700 w702] -> w3
    tunnel: w1 -> [w700 w702]
    frame No Error {
      n9 = Unbundle By Name(w700) -> ("Image Path"=w696:string, "Last Image"=w697:string)
      n10 = local read "Header Contents"() -> (w14:T1)
      n11 = Concatenate Strings(w696, w697) -> (w695:string)
      n12 = String To Path(string=w695) -> (path=w692:path)
      n13 = Unbundle By Name(w14) -> ("FILENAME"=w691:string[], "OBSERVER"=w678:string[], "PROGRID"=w668:string[], "OBJECT"=w643:string[], "NIGHTDIR"=w642:string[], "CHANNEL"=w641:string[], "INSTRUME"=w589:string[], "NEXPSEQ"=w588:string[], "SEQINDEX"=w587:string[], "OBSTYPE"=w586:string[], "READMOD"=w585:string[], "SHUTTER"=w584:string[], "OPENSHT"=w487:string[], "CLOSESHT"=w486:string[], "GAIN"=w485:string[], "GAINERR"=w484:string[], "RDNOISE"=w483:string[], "RNOISERR"=w482:string[], "SKYFIBER"=w481:string[], "CALFIBER"=w480:string[], "UTDATE"=w479:string[], "LOCTIME"=w478:string[], "MJD"=w477:string[], "OBSLON"=w476:string[], "OBSLAT"=w347:string[], "OBSALT"=w346:string[], "EXPTIME"=w345:string[], "TELRA"=w344:string[], "TELDEC"=w343:string[], "RA"=w342:string[], "DEC"=w341:string[], "RA_DEG"=w340:string[], "DEC_DEG"=w339:string[], "EPOCH"=w338:string[], "HA"=w337:string[], "HAD"=w336:string[], "AIRMASS"=w335:string[], "AMSTART"=w334:string[], "AMEND"=w333:string[], "XOFFSET"=w332:string[], "YOFFSET"=w211:string[], "PA"=w210:string[], "CAMFOC"=w209:string[], "TELFOC"=w208:string[], "TCSUT"=w207:string[], "MOONDIST"=w206:string[], "MOONALT"=w205:string[], "MONNPHAS"=w204:string[], "ADC"=w203:string[], "ADCSPPED"=w202:string[], "CALMIRR"=w201:string[], "GUIDING"=w200:string[], "GUIDTEXP"=w199:string[], "GUIDFREQ"=w198:string[], "GUIDOBJX"=w197:string[], "GUIDOBJY"=w76:string[], "AVGYCORR"=w75:string[], "AVGXCORR"=w74:string[], "GFOCUS"=w73:string[], "THARLAMP"=w72:string[], "HALLAMP"=w71:string[], "AGITATOR"=w70:string[], "THARMIRR"=w69:string[], "DSTATUS"=w68:string[], "DTEMP"=w67:string[], "DHUM"=w66:string[], "DLAMP"=w65:string[], "DFLAT"=w64:string[], "TEMPEXT"=w63:string[], "PRESSURE"=w62:string[], "HUMIDITY"=w21:string[], "WINDDIR"=w20:string[], "WSPEED"=w19:string[], "TCSST"=w18:string[], "DPOS"=w17:string[])
      n14 = call <userlib>:"gfitsio-open-create-replace-file.vi"("error in (no error)"=w701, "function (open)"=T2."open", "file path (dialog if empty)"=w692) -> ("error out"=w698:errorcluster, "gfits refnum"=w694:T3)  [unwired: 6 in, 1 out]
      n15 = Index Array(array=w691, index #1=0 ("index"), index #2=1 ("index"), index #3=2 ("index")) -> (element #1=w687:string, element #2=w686:string, element #3=w685:string)
      n16 = call <userlib>:"gfitsio-get-hdu-list.vi"("error in (no error)"=w698, "gfits refnum"=w694) -> ("error out"=w638:errorcluster, "dup gfits refnum"=w675:T3)  [unwired: 6 in, 2 out]
      n17 = Index Array(array=w678, index #1=0 ("index"), index #2=1 ("index"), index #3=2 ("index")) -> (element #1=w682:string, element #2=w683:string, element #3=w684:string)
      n18 = call-poly <userlib>:"gfitsio-write-key.vi"("comment"=w685, "keyname"=w687, "error in (no error)"=w638, "value"=w686, "gfits refnum"=w675) -> ("error out"=w677:errorcluster, "dup gfits refnum"=w676:T3)  [unwired: 5 in]
      n19 = Index Array(array=w668, index #1=0 ("index"), index #2=1 ("index"), index #3=2 ("index")) -> (element #1=w671:string, element #2=w670:string, element #3=w669:string)
      n20 = call-poly <userlib>:"gfitsio-write-key.vi"("comment"=w684, "keyname"=w682, "error in (no error)"=w677, "value"=w683, "gfits refnum"=w676) -> ("error out"=w667:errorcluster, "dup gfits refnum"=w666:T3)  [unwired: 5 in]
      n21 = Index Array(array=w643, index #1=0 ("index"), index #2=1 ("index"), index #3=2 ("index")) -> (element #1=w647:string, element #2=w648:string, element #3=w649:string)
      n22 = call-poly <userlib>:"gfitsio-write-key.vi"("comment"=w669, "keyname"=w671, "error in (no error)"=w667, "value"=w670, "gfits refnum"=w666) -> ("error out"=w640:errorcluster, "dup gfits refnum"=w639:T3)  [unwired: 5 in]
      n23 = Index Array(array=w642, index #1=0 ("index"), index #2=1 ("index"), index #3=2 ("index")) -> (element #1=w652:string, element #2=w651:string, element #3=w650:string)
      n24 = call-poly <userlib>:"gfitsio-write-key.vi"("comment"=w649, "keyname"=w647, "error in (no error)"=w640, "value"=w648, "gfits refnum"=w639) -> ("error out"=w656:errorcluster, "dup gfits refnum"=w657:T3)  [unwired: 5 in]
      n25 = Index Array(array=w641, index #1=0 ("index"), index #2=1 ("index"), index #3=2 ("index")) -> (element #1=w661:string, element #2=w662:string, element #3=w663:string)
      n26 = call-poly <userlib>:"gfitsio-write-key.vi"("comment"=w650, "keyname"=w652, "error in (no error)"=w656, "value"=w651, "gfits refnum"=w657) -> ("error out"=w664:errorcluster, "dup gfits refnum"=w665:T3)  [unwired: 5 in]
      n27 = Index Array(array=w589, index #1=0 ("index"), index #2=1 ("index"), index #3=2 ("index")) -> (element #1=w595:string, element #2=w596:string, element #3=w597:string)
      n28 = call-poly <userlib>:"gfitsio-write-key.vi"("comment"=w663, "keyname"=w661, "error in (no error)"=w664, "value"=w662, "gfits refnum"=w665) -> ("error out"=w591:errorcluster, "dup gfits refnum"=w590:T3)  [unwired: 5 in]
      n29 = Index Array(array=w588, index #1=0 ("index"), index #2=1 ("index"), index #3=2 ("index")) -> (element #1=w600:string, element #2=w599:string, element #3=w598:string)
      n30 = call-poly <userlib>:"gfitsio-write-key.vi"("comment"=w597, "keyname"=w595, "error in (no error)"=w591, "value"=w596, "gfits refnum"=w590) -> ("error out"=w604:errorcluster, "dup gfits refnum"=w605:T3)  [unwired: 5 in]
      n31 = Index Array(array=w587, index #1=0 ("index"), index #2=1 ("index"), index #3=2 ("index")) -> (element #1=w609:string, element #2=w610:string, element #3=w611:string)
      n32 = call-poly <userlib>:"gfitsio-write-key.vi"("comment"=w598, "keyname"=w600, "error in (no error)"=w604, "value"=w599, "gfits refnum"=w605) -> ("error out"=w612:errorcluster, "dup gfits refnum"=w613:T3)  [unwired: 5 in]
      n33 = Index Array(array=w586, index #1=0 ("index"), index #2=1 ("index"), index #3=2 ("index")) -> (element #1=w632:string, element #2=w631:string, element #3=w630:string)
      n34 = call-poly <userlib>:"gfitsio-write-key.vi"("comment"=w611, "keyname"=w609, "error in (no error)"=w612, "value"=w610, "gfits refnum"=w613) -> ("error out"=w636:errorcluster, "dup gfits refnum"=w637:T3)  [unwired: 5 in]
      n35 = Index Array(array=w585, index #1=0 ("index"), index #2=1 ("index"), index #3=2 ("index")) -> (element #1=w627:string, element #2=w628:string, element #3=w629:string)
      n36 = call-poly <userlib>:"gfitsio-write-key.vi"("comment"=w630, "keyname"=w632, "error in (no error)"=w636, "value"=w631, "gfits refnum"=w637) -> ("error out"=w623:errorcluster, "dup gfits refnum"=w622:T3)  [unwired: 5 in]
      n37 = Index Array(array=w584, index #1=0 ("index"), index #2=1 ("index"), index #3=2 ("index")) -> (element #1=w618:string, element #2=w617:string, element #3=w616:string)
      n38 = call-poly <userlib>:"gfitsio-write-key.vi"("comment"=w629, "keyname"=w627, "error in (no error)"=w623, "value"=w628, "gfits refnum"=w622) -> ("error out"=w615:errorcluster, "dup gfits refnum"=w614:T3)  [unwired: 5 in]
      n39 = Index Array(array=w487, index #1=0 ("index"), index #2=1 ("index"), index #3=2 ("index")) -> (element #1=w493:string, element #2=w494:string, element #3=w495:string)
      n40 = call-poly <userlib>:"gfitsio-write-key.vi"("comment"=w616, "keyname"=w618, "error in (no error)"=w615, "value"=w617, "gfits refnum"=w614) -> ("error out"=w489:errorcluster, "dup gfits refnum"=w488:T3)  [unwired: 5 in]
      n41 = Index Array(array=w486, index #1=0 ("index"), index #2=1 ("index"), index #3=2 ("index")) -> (element #1=w498:string, element #2=w497:string, element #3=w496:string)
      n42 = call-poly <userlib>:"gfitsio-write-key.vi"("comment"=w495, "keyname"=w493, "error in (no error)"=w489, "value"=w494, "gfits refnum"=w488) -> ("error out"=w502:errorcluster, "dup gfits refnum"=w503:T3)  [unwired: 5 in]
      n43 = Index Array(array=w485, index #1=0 ("index"), index #2=1 ("index"), index #3=2 ("index")) -> (element #1=w507:string, element #2=w508:string, element #3=w509:string)
      n44 = call-poly <userlib>:"gfitsio-write-key.vi"("comment"=w496, "keyname"=w498, "error in (no error)"=w502, "value"=w497, "gfits refnum"=w503) -> ("error out"=w510:errorcluster, "dup gfits refnum"=w511:T3)  [unwired: 5 in]
      n45 = Index Array(array=w484, index #1=0 ("index"), index #2=1 ("index"), index #3=2 ("index")) -> (element #1=w530:string, element #2=w529:string, element #3=w528:string)
      n46 = call-poly <userlib>:"gfitsio-write-key.vi"("comment"=w509, "keyname"=w507, "error in (no error)"=w510, "value"=w508, "gfits refnum"=w511) -> ("error out"=w534:errorcluster, "dup gfits refnum"=w535:T3)  [unwired: 5 in]
      n47 = Index Array(array=w483, index #1=0 ("index"), index #2=1 ("index"), index #3=2 ("index")) -> (element #1=w525:string, element #2=w526:string, element #3=w527:string)
      n48 = call-poly <userlib>:"gfitsio-write-key.vi"("comment"=w528, "keyname"=w530, "error in (no error)"=w534, "value"=w529, "gfits refnum"=w535) -> ("error out"=w521:errorcluster, "dup gfits refnum"=w520:T3)  [unwired: 5 in]
      n49 = Index Array(array=w482, index #1=0 ("index"), index #2=1 ("index"), index #3=2 ("index")) -> (element #1=w516:string, element #2=w515:string, element #3=w514:string)
      n50 = call-poly <userlib>:"gfitsio-write-key.vi"("comment"=w527, "keyname"=w525, "error in (no error)"=w521, "value"=w526, "gfits refnum"=w520) -> ("error out"=w513:errorcluster, "dup gfits refnum"=w512:T3)  [unwired: 5 in]
      n51 = Index Array(array=w481, index #1=0 ("index"), index #2=1 ("index"), index #3=2 ("index")) -> (element #1=w578:string, element #2=w577:string, element #3=w576:string)
      n52 = call-poly <userlib>:"gfitsio-write-key.vi"("comment"=w514, "keyname"=w516, "error in (no error)"=w513, "value"=w515, "gfits refnum"=w512) -> ("error out"=w582:errorcluster, "dup gfits refnum"=w583:T3)  [unwired: 5 in]
      n53 = Index Array(array=w480, index #1=0 ("index"), index #2=1 ("index"), index #3=2 ("index")) -> (element #1=w573:string, element #2=w574:string, element #3=w575:string)
      n54 = call-poly <userlib>:"gfitsio-write-key.vi"("comment"=w576, "keyname"=w578, "error in (no error)"=w582, "value"=w577, "gfits refnum"=w583) -> ("error out"=w569:errorcluster, "dup gfits refnum"=w568:T3)  [unwired: 5 in]
      n55 = Index Array(array=w479, index #1=0 ("index"), index #2=1 ("index"), index #3=2 ("index")) -> (element #1=w564:string, element #2=w563:string, element #3=w562:string)
      n56 = call-poly <userlib>:"gfitsio-write-key.vi"("comment"=w575, "keyname"=w573, "error in (no error)"=w569, "value"=w574, "gfits refnum"=w568) -> ("error out"=w561:errorcluster, "dup gfits refnum"=w560:T3)  [unwired: 5 in]
      n57 = Index Array(array=w478, index #1=0 ("index"), index #2=1 ("index"), index #3=2 ("index")) -> (element #1=w541:string, element #2=w542:string, element #3=w543:string)
      n58 = call-poly <userlib>:"gfitsio-write-key.vi"("comment"=w562, "keyname"=w564, "error in (no error)"=w561, "value"=w563, "gfits refnum"=w560) -> ("error out"=w537:errorcluster, "dup gfits refnum"=w536:T3)  [unwired: 5 in]
      n59 = Index Array(array=w477, index #1=0 ("index"), index #2=1 ("index"), index #3=2 ("index")) -> (element #1=w546:string, element #2=w545:string, element #3=w544:string)
      n60 = call-poly <userlib>:"gfitsio-write-key.vi"("comment"=w543, "keyname"=w541, "error in (no error)"=w537, "value"=w542, "gfits refnum"=w536) -> ("error out"=w550:errorcluster, "dup gfits refnum"=w551:T3)  [unwired: 5 in]
      n61 = Index Array(array=w476, index #1=0 ("index"), index #2=1 ("index"), index #3=2 ("index")) -> (element #1=w555:string, element #2=w556:string, element #3=w557:string)
      n62 = call-poly <userlib>:"gfitsio-write-key.vi"("comment"=w544, "keyname"=w546, "error in (no error)"=w550, "value"=w545, "gfits refnum"=w551) -> ("error out"=w558:errorcluster, "dup gfits refnum"=w559:T3)  [unwired: 5 in]
      n63 = Index Array(array=w347, index #1=0 ("index"), index #2=1 ("index"), index #3=2 ("index")) -> (element #1=w376:string, element #2=w375:string, element #3=w374:string)
      n64 = call-poly <userlib>:"gfitsio-write-key.vi"("comment"=w557, "keyname"=w555, "error in (no error)"=w558, "value"=w556, "gfits refnum"=w559) -> ("error out"=w349:errorcluster, "dup gfits refnum"=w348:T3)  [unwired: 5 in]
      n65 = Index Array(array=w346, index #1=0 ("index"), index #2=1 ("index"), index #3=2 ("index")) -> (element #1=w355:string, element #2=w356:string, element #3=w357:string)
      n66 = call-poly <userlib>:"gfitsio-write-key.vi"("comment"=w374, "keyname"=w376, "error in (no error)"=w349, "value"=w375, "gfits refnum"=w348) -> ("error out"=w351:errorcluster, "dup gfits refnum"=w350:T3)  [unwired: 5 in]
      n67 = Index Array(array=w345, index #1=0 ("index"), index #2=1 ("index"), index #3=2 ("index")) -> (element #1=w360:string, element #2=w359:string, element #3=w358:string)
      n68 = call-poly <userlib>:"gfitsio-write-key.vi"("comment"=w357, "keyname"=w355, "error in (no error)"=w351, "value"=w356, "gfits refnum"=w350) -> ("error out"=w364:errorcluster, "dup gfits refnum"=w365:T3)  [unwired: 5 in]
      n69 = Index Array(array=w344, index #1=0 ("index"), index #2=1 ("index"), index #3=2 ("index")) -> (element #1=w369:string, element #2=w370:string, element #3=w371:string)
      n70 = call-poly <userlib>:"gfitsio-write-key.vi"("comment"=w358, "keyname"=w360, "error in (no error)"=w364, "value"=w359, "gfits refnum"=w365) -> ("error out"=w372:errorcluster, "dup gfits refnum"=w373:T3)  [unwired: 5 in]
      n71 = Index Array(array=w343, index #1=0 ("index"), index #2=1 ("index"), index #3=2 ("index")) -> (element #1=w470:string, element #2=w469:string, element #3=w468:string)
      n72 = call-poly <userlib>:"gfitsio-write-key.vi"("comment"=w371, "keyname"=w369, "error in (no error)"=w372, "value"=w370, "gfits refnum"=w373) -> ("error out"=w474:errorcluster, "dup gfits refnum"=w475:T3)  [unwired: 5 in]
      n73 = Index Array(array=w342, index #1=0 ("index"), index #2=1 ("index"), index #3=2 ("index")) -> (element #1=w465:string, element #2=w466:string, element #3=w467:string)
      n74 = call-poly <userlib>:"gfitsio-write-key.vi"("comment"=w468, "keyname"=w470, "error in (no error)"=w474, "value"=w469, "gfits refnum"=w475) -> ("error out"=w461:errorcluster, "dup gfits refnum"=w460:T3)  [unwired: 5 in]
      n75 = Index Array(array=w341, index #1=0 ("index"), index #2=1 ("index"), index #3=2 ("index")) -> (element #1=w456:string, element #2=w455:string, element #3=w454:string)
      n76 = call-poly <userlib>:"gfitsio-write-key.vi"("comment"=w467, "keyname"=w465, "error in (no error)"=w461, "value"=w466, "gfits refnum"=w460) -> ("error out"=w453:errorcluster, "dup gfits refnum"=w452:T3)  [unwired: 5 in]
      n77 = Index Array(array=w340, index #1=0 ("index"), index #2=1 ("index"), index #3=2 ("index")) -> (element #1=w433:string, element #2=w434:string, element #3=w435:string)
      n78 = call-poly <userlib>:"gfitsio-write-key.vi"("comment"=w454, "keyname"=w456, "error in (no error)"=w453, "value"=w455, "gfits refnum"=w452) -> ("error out"=w429:errorcluster, "dup gfits refnum"=w428:T3)  [unwired: 5 in]
      n79 = Index Array(array=w339, index #1=0 ("index"), index #2=1 ("index"), index #3=2 ("index")) -> (element #1=w438:string, element #2=w437:string, element #3=w436:string)
      n80 = call-poly <userlib>:"gfitsio-write-key.vi"("comment"=w435, "keyname"=w433, "error in (no error)"=w429, "value"=w434, "gfits refnum"=w428) -> ("error out"=w442:errorcluster, "dup gfits refnum"=w443:T3)  [unwired: 5 in]
      n81 = Index Array(array=w338, index #1=0 ("index"), index #2=1 ("index"), index #3=2 ("index")) -> (element #1=w447:string, element #2=w448:string, element #3=w449:string)
      n82 = call-poly <userlib>:"gfitsio-write-key.vi"("comment"=w436, "keyname"=w438, "error in (no error)"=w442, "value"=w437, "gfits refnum"=w443) -> ("error out"=w450:errorcluster, "dup gfits refnum"=w451:T3)  [unwired: 5 in]
      n83 = Index Array(array=w337, index #1=0 ("index"), index #2=1 ("index"), index #3=2 ("index")) -> (element #1=w385:string, element #2=w386:string, element #3=w387:string)
      n84 = call-poly <userlib>:"gfitsio-write-key.vi"("comment"=w449, "keyname"=w447, "error in (no error)"=w450, "value"=w448, "gfits refnum"=w451) -> ("error out"=w381:errorcluster, "dup gfits refnum"=w380:T3)  [unwired: 5 in]
      n85 = Index Array(array=w336, index #1=0 ("index"), index #2=1 ("index"), index #3=2 ("index")) -> (element #1=w390:string, element #2=w389:string, element #3=w388:string)
      n86 = call-poly <userlib>:"gfitsio-write-key.vi"("comment"=w387, "keyname"=w385, "error in (no error)"=w381, "value"=w386, "gfits refnum"=w380) -> ("error out"=w394:errorcluster, "dup gfits refnum"=w395:T3)  [unwired: 5 in]
      n87 = Index Array(array=w335, index #1=0 ("index"), index #2=1 ("index"), index #3=2 ("index")) -> (element #1=w399:string, element #2=w400:string, element #3=w401:string)
      n88 = call-poly <userlib>:"gfitsio-write-key.vi"("comment"=w388, "keyname"=w390, "error in (no error)"=w394, "value"=w389, "gfits refnum"=w395) -> ("error out"=w402:errorcluster, "dup gfits refnum"=w403:T3)  [unwired: 5 in]
      n89 = Index Array(array=w334, index #1=0 ("index"), index #2=1 ("index"), index #3=2 ("index")) -> (element #1=w422:string, element #2=w421:string, element #3=w420:string)
      n90 = call-poly <userlib>:"gfitsio-write-key.vi"("comment"=w401, "keyname"=w399, "error in (no error)"=w402, "value"=w400, "gfits refnum"=w403) -> ("error out"=w426:errorcluster, "dup gfits refnum"=w427:T3)  [unwired: 5 in]
      n91 = Index Array(array=w333, index #1=0 ("index"), index #2=1 ("index"), index #3=2 ("index")) -> (element #1=w417:string, element #2=w418:string, element #3=w419:string)
      n92 = call-poly <userlib>:"gfitsio-write-key.vi"("comment"=w420, "keyname"=w422, "error in (no error)"=w426, "value"=w421, "gfits refnum"=w427) -> ("error out"=w413:errorcluster, "dup gfits refnum"=w412:T3)  [unwired: 5 in]
      n93 = Index Array(array=w332, index #1=0 ("index"), index #2=1 ("index"), index #3=2 ("index")) -> (element #1=w408:string, element #2=w407:string, element #3=w406:string)
      n94 = call-poly <userlib>:"gfitsio-write-key.vi"("comment"=w419, "keyname"=w417, "error in (no error)"=w413, "value"=w418, "gfits refnum"=w412) -> ("error out"=w405:errorcluster, "dup gfits refnum"=w404:T3)  [unwired: 5 in]
      n95 = Index Array(array=w211, index #1=0 ("index"), index #2=1 ("index"), index #3=2 ("index")) -> (element #1=w328:string, element #2=w327:string, element #3=w326:string)
      n96 = call-poly <userlib>:"gfitsio-write-key.vi"("comment"=w406, "keyname"=w408, "error in (no error)"=w405, "value"=w407, "gfits refnum"=w404) -> ("error out"=w213:errorcluster, "dup gfits refnum"=w212:T3)  [unwired: 5 in]
      n97 = Index Array(array=w210, index #1=0 ("index"), index #2=1 ("index"), index #3=2 ("index")) -> (element #1=w323:string, element #2=w324:string, element #3=w325:string)
      n98 = call-poly <userlib>:"gfitsio-write-key.vi"("comment"=w326, "keyname"=w328, "error in (no error)"=w213, "value"=w327, "gfits refnum"=w212) -> ("error out"=w319:errorcluster, "dup gfits refnum"=w318:T3)  [unwired: 5 in]
      n99 = Index Array(array=w209, index #1=0 ("index"), index #2=1 ("index"), index #3=2 ("index")) -> (element #1=w314:string, element #2=w313:string, element #3=w312:string)
      n100 = call-poly <userlib>:"gfitsio-write-key.vi"("comment"=w325, "keyname"=w323, "error in (no error)"=w319, "value"=w324, "gfits refnum"=w318) -> ("error out"=w311:errorcluster, "dup gfits refnum"=w310:T3)  [unwired: 5 in]
      n101 = Index Array(array=w208, index #1=0 ("index"), index #2=1 ("index"), index #3=2 ("index")) -> (element #1=w219:string, element #2=w220:string, element #3=w221:string)
      n102 = call-poly <userlib>:"gfitsio-write-key.vi"("comment"=w312, "keyname"=w314, "error in (no error)"=w311, "value"=w313, "gfits refnum"=w310) -> ("error out"=w215:errorcluster, "dup gfits refnum"=w214:T3)  [unwired: 5 in]
      n103 = Index Array(array=w207, index #1=0 ("index"), index #2=1 ("index"), index #3=2 ("index")) -> (element #1=w224:string, element #2=w223:string, element #3=w222:string)
      n104 = call-poly <userlib>:"gfitsio-write-key.vi"("comment"=w221, "keyname"=w219, "error in (no error)"=w215, "value"=w220, "gfits refnum"=w214) -> ("error out"=w228:errorcluster, "dup gfits refnum"=w229:T3)  [unwired: 5 in]
      n105 = Index Array(array=w206, index #1=0 ("index"), index #2=1 ("index"), index #3=2 ("index")) -> (element #1=w233:string, element #2=w234:string, element #3=w235:string)
      n106 = call-poly <userlib>:"gfitsio-write-key.vi"("comment"=w222, "keyname"=w224, "error in (no error)"=w228, "value"=w223, "gfits refnum"=w229) -> ("error out"=w236:errorcluster, "dup gfits refnum"=w237:T3)  [unwired: 5 in]
      n107 = Index Array(array=w205, index #1=0 ("index"), index #2=1 ("index"), index #3=2 ("index")) -> (element #1=w256:string, element #2=w255:string, element #3=w254:string)
      n108 = call-poly <userlib>:"gfitsio-write-key.vi"("comment"=w235, "keyname"=w233, "error in (no error)"=w236, "value"=w234, "gfits refnum"=w237) -> ("error out"=w260:errorcluster, "dup gfits refnum"=w261:T3)  [unwired: 5 in]
      n109 = Index Array(array=w204, index #1=0 ("index"), index #2=1 ("index"), index #3=2 ("index")) -> (element #1=w251:string, element #2=w252:string, element #3=w253:string)
      n110 = call-poly <userlib>:"gfitsio-write-key.vi"("comment"=w254, "keyname"=w256, "error in (no error)"=w260, "value"=w255, "gfits refnum"=w261) -> ("error out"=w247:errorcluster, "dup gfits refnum"=w246:T3)  [unwired: 5 in]
      n111 = Index Array(array=w203, index #1=0 ("index"), index #2=1 ("index"), index #3=2 ("index")) -> (element #1=w242:string, element #2=w241:string, element #3=w240:string)
      n112 = call-poly <userlib>:"gfitsio-write-key.vi"("comment"=w253, "keyname"=w251, "error in (no error)"=w247, "value"=w252, "gfits refnum"=w246) -> ("error out"=w239:errorcluster, "dup gfits refnum"=w238:T3)  [unwired: 5 in]
      n113 = Index Array(array=w202, index #1=0 ("index"), index #2=1 ("index"), index #3=2 ("index")) -> (element #1=w304:string, element #2=w303:string, element #3=w302:string)
      n114 = call-poly <userlib>:"gfitsio-write-key.vi"("comment"=w240, "keyname"=w242, "error in (no error)"=w239, "value"=w241, "gfits refnum"=w238) -> ("error out"=w308:errorcluster, "dup gfits refnum"=w309:T3)  [unwired: 5 in]
      n115 = Index Array(array=w201, index #1=0 ("index"), index #2=1 ("index"), index #3=2 ("index")) -> (element #1=w299:string, element #2=w300:string, element #3=w301:string)
      n116 = call-poly <userlib>:"gfitsio-write-key.vi"("comment"=w302, "keyname"=w304, "error in (no error)"=w308, "value"=w303, "gfits refnum"=w309) -> ("error out"=w295:errorcluster, "dup gfits refnum"=w294:T3)  [unwired: 5 in]
      n117 = Index Array(array=w200, index #1=0 ("index"), index #2=1 ("index"), index #3=2 ("index")) -> (element #1=w290:string, element #2=w289:string, element #3=w288:string)
      n118 = call-poly <userlib>:"gfitsio-write-key.vi"("comment"=w301, "keyname"=w299, "error in (no error)"=w295, "value"=w300, "gfits refnum"=w294) -> ("error out"=w287:errorcluster, "dup gfits refnum"=w286:T3)  [unwired: 5 in]
      n119 = Index Array(array=w199, index #1=0 ("index"), index #2=1 ("index"), index #3=2 ("index")) -> (element #1=w267:string, element #2=w268:string, element #3=w269:string)
      n120 = call-poly <userlib>:"gfitsio-write-key.vi"("comment"=w288, "keyname"=w290, "error in (no error)"=w287, "value"=w289, "gfits refnum"=w286) -> ("error out"=w263:errorcluster, "dup gfits refnum"=w262:T3)  [unwired: 5 in]
      n121 = Index Array(array=w198, index #1=0 ("index"), index #2=1 ("index"), index #3=2 ("index")) -> (element #1=w272:string, element #2=w271:string, element #3=w270:string)
      n122 = call-poly <userlib>:"gfitsio-write-key.vi"("comment"=w269, "keyname"=w267, "error in (no error)"=w263, "value"=w268, "gfits refnum"=w262) -> ("error out"=w276:errorcluster, "dup gfits refnum"=w277:T3)  [unwired: 5 in]
      n123 = Index Array(array=w197, index #1=0 ("index"), index #2=1 ("index"), index #3=2 ("index")) -> (element #1=w281:string, element #2=w282:string, element #3=w283:string)
      n124 = call-poly <userlib>:"gfitsio-write-key.vi"("comment"=w270, "keyname"=w272, "error in (no error)"=w276, "value"=w271, "gfits refnum"=w277) -> ("error out"=w284:errorcluster, "dup gfits refnum"=w285:T3)  [unwired: 5 in]
      n125 = Index Array(array=w76, index #1=0 ("index"), index #2=1 ("index"), index #3=2 ("index")) -> (element #1=w82:string, element #2=w83:string, element #3=w84:string)
      n126 = call-poly <userlib>:"gfitsio-write-key.vi"("comment"=w283, "keyname"=w281, "error in (no error)"=w284, "value"=w282, "gfits refnum"=w285) -> ("error out"=w78:errorcluster, "dup gfits refnum"=w77:T3)  [unwired: 5 in]
      n127 = Index Array(array=w75, index #1=0 ("index"), index #2=1 ("index"), index #3=2 ("index")) -> (element #1=w87:string, element #2=w86:string, element #3=w85:string)
      n128 = call-poly <userlib>:"gfitsio-write-key.vi"("comment"=w84, "keyname"=w82, "error in (no error)"=w78, "value"=w83, "gfits refnum"=w77) -> ("error out"=w91:errorcluster, "dup gfits refnum"=w92:T3)  [unwired: 5 in]
      n129 = Index Array(array=w74, index #1=0 ("index"), index #2=1 ("index"), index #3=2 ("index")) -> (element #1=w96:string, element #2=w97:string, element #3=w98:string)
      n130 = call-poly <userlib>:"gfitsio-write-key.vi"("comment"=w85, "keyname"=w87, "error in (no error)"=w91, "value"=w86, "gfits refnum"=w92) -> ("error out"=w99:errorcluster, "dup gfits refnum"=w100:T3)  [unwired: 5 in]
      n131 = Index Array(array=w73, index #1=0 ("index"), index #2=1 ("index"), index #3=2 ("index")) -> (element #1=w191:string, element #2=w190:string, element #3=w189:string)
      n132 = call-poly <userlib>:"gfitsio-write-key.vi"("comment"=w98, "keyname"=w96, "error in (no error)"=w99, "value"=w97, "gfits refnum"=w100) -> ("error out"=w195:errorcluster, "dup gfits refnum"=w196:T3)  [unwired: 5 in]
      n133 = Index Array(array=w72, index #1=0 ("index"), index #2=1 ("index"), index #3=2 ("index")) -> (element #1=w186:string, element #2=w187:string, element #3=w188:string)
      n134 = call-poly <userlib>:"gfitsio-write-key.vi"("comment"=w189, "keyname"=w191, "error in (no error)"=w195, "value"=w190, "gfits refnum"=w196) -> ("error out"=w182:errorcluster, "dup gfits refnum"=w181:T3)  [unwired: 5 in]
      n135 = Index Array(array=w71, index #1=0 ("index"), index #2=1 ("index"), index #3=2 ("index")) -> (element #1=w177:string, element #2=w176:string, element #3=w175:string)
      n136 = call-poly <userlib>:"gfitsio-write-key.vi"("comment"=w188, "keyname"=w186, "error in (no error)"=w182, "value"=w187, "gfits refnum"=w181) -> ("error out"=w174:errorcluster, "dup gfits refnum"=w173:T3)  [unwired: 5 in]
      n137 = Index Array(array=w70, index #1=0 ("index"), index #2=1 ("index"), index #3=2 ("index")) -> (element #1=w154:string, element #2=w155:string, element #3=w156:string)
      n138 = call-poly <userlib>:"gfitsio-write-key.vi"("comment"=w175, "keyname"=w177, "error in (no error)"=w174, "value"=w176, "gfits refnum"=w173) -> ("error out"=w150:errorcluster, "dup gfits refnum"=w149:T3)  [unwired: 5 in]
      n139 = Index Array(array=w69, index #1=0 ("index"), index #2=1 ("index"), index #3=2 ("index")) -> (element #1=w159:string, element #2=w158:string, element #3=w157:string)
      n140 = call-poly <userlib>:"gfitsio-write-key.vi"("comment"=w156, "keyname"=w154, "error in (no error)"=w150, "value"=w155, "gfits refnum"=w149) -> ("error out"=w163:errorcluster, "dup gfits refnum"=w164:T3)  [unwired: 5 in]
      n141 = Index Array(array=w68, index #1=0 ("index"), index #2=1 ("index"), index #3=2 ("index")) -> (element #1=w168:string, element #2=w169:string, element #3=w170:string)
      n142 = call-poly <userlib>:"gfitsio-write-key.vi"("comment"=w157, "keyname"=w159, "error in (no error)"=w163, "value"=w158, "gfits refnum"=w164) -> ("error out"=w171:errorcluster, "dup gfits refnum"=w172:T3)  [unwired: 5 in]
      n143 = Index Array(array=w67, index #1=0 ("index"), index #2=1 ("index"), index #3=2 ("index")) -> (element #1=w106:string, element #2=w107:string, element #3=w108:string)
      n144 = call-poly <userlib>:"gfitsio-write-key.vi"("comment"=w170, "keyname"=w168, "error in (no error)"=w171, "value"=w169, "gfits refnum"=w172) -> ("error out"=w102:errorcluster, "dup gfits refnum"=w101:T3)  [unwired: 5 in]
      n145 = Index Array(array=w66, index #1=0 ("index"), index #2=1 ("index"), index #3=2 ("index")) -> (element #1=w111:string, element #2=w110:string, element #3=w109:string)
      n146 = call-poly <userlib>:"gfitsio-write-key.vi"("comment"=w108, "keyname"=w106, "error in (no error)"=w102, "value"=w107, "gfits refnum"=w101) -> ("error out"=w115:errorcluster, "dup gfits refnum"=w116:T3)  [unwired: 5 in]
      n147 = Index Array(array=w65, index #1=0 ("index"), index #2=1 ("index"), index #3=2 ("index")) -> (element #1=w120:string, element #2=w121:string, element #3=w122:string)
      n148 = call-poly <userlib>:"gfitsio-write-key.vi"("comment"=w109, "keyname"=w111, "error in (no error)"=w115, "value"=w110, "gfits refnum"=w116) -> ("error out"=w123:errorcluster, "dup gfits refnum"=w124:T3)  [unwired: 5 in]
      n149 = Index Array(array=w64, index #1=0 ("index"), index #2=1 ("index"), index #3=2 ("index")) -> (element #1=w143:string, element #2=w142:string, element #3=w141:string)
      n150 = call-poly <userlib>:"gfitsio-write-key.vi"("comment"=w122, "keyname"=w120, "error in (no error)"=w123, "value"=w121, "gfits refnum"=w124) -> ("error out"=w147:errorcluster, "dup gfits refnum"=w148:T3)  [unwired: 5 in]
      n151 = Index Array(array=w63, index #1=0 ("index"), index #2=1 ("index"), index #3=2 ("index")) -> (element #1=w138:string, element #2=w139:string, element #3=w140:string)
      n152 = call-poly <userlib>:"gfitsio-write-key.vi"("comment"=w141, "keyname"=w143, "error in (no error)"=w147, "value"=w142, "gfits refnum"=w148) -> ("error out"=w134:errorcluster, "dup gfits refnum"=w133:T3)  [unwired: 5 in]
      n153 = Index Array(array=w62, index #1=0 ("index"), index #2=1 ("index"), index #3=2 ("index")) -> (element #1=w129:string, element #2=w128:string, element #3=w127:string)
      n154 = call-poly <userlib>:"gfitsio-write-key.vi"("comment"=w140, "keyname"=w138, "error in (no error)"=w134, "value"=w139, "gfits refnum"=w133) -> ("error out"=w126:errorcluster, "dup gfits refnum"=w125:T3)  [unwired: 5 in]
      n155 = Index Array(array=w21, index #1=0 ("index"), index #2=1 ("index"), index #3=2 ("index")) -> (element #1=w42:string, element #2=w41:string, element #3=w40:string)
      n156 = call-poly <userlib>:"gfitsio-write-key.vi"("comment"=w127, "keyname"=w129, "error in (no error)"=w126, "value"=w128, "gfits refnum"=w125) -> ("error out"=w23:errorcluster, "dup gfits refnum"=w22:T3)  [unwired: 5 in]
      n157 = Index Array(array=w20, index #1=0 ("index"), index #2=1 ("index"), index #3=2 ("index")) -> (element #1=w37:string, element #2=w38:string, element #3=w39:string)
      n158 = call-poly <userlib>:"gfitsio-write-key.vi"("comment"=w40, "keyname"=w42, "error in (no error)"=w23, "value"=w41, "gfits refnum"=w22) -> ("error out"=w33:errorcluster, "dup gfits refnum"=w32:T3)  [unwired: 5 in]
      n159 = Index Array(array=w19, index #1=0 ("index"), index #2=1 ("index"), index #3=2 ("index")) -> (element #1=w28:string, element #2=w27:string, element #3=w26:string)
      n160 = call-poly <userlib>:"gfitsio-write-key.vi"("comment"=w39, "keyname"=w37, "error in (no error)"=w33, "value"=w38, "gfits refnum"=w32) -> ("error out"=w25:errorcluster, "dup gfits refnum"=w24:T3)  [unwired: 5 in]
      n161 = Index Array(array=w18, index #1=0 ("index"), index #2=1 ("index"), index #3=2 ("index")) -> (element #1=w56:string, element #2=w55:string, element #3=w54:string)
      n162 = call-poly <userlib>:"gfitsio-write-key.vi"("comment"=w26, "keyname"=w28, "error in (no error)"=w25, "value"=w27, "gfits refnum"=w24) -> ("error out"=w60:errorcluster, "dup gfits refnum"=w61:T3)  [unwired: 5 in]
      n163 = Index Array(array=w17, index #1=0 ("index"), index #2=1 ("index"), index #3=2 ("index")) -> (element #1=w51:string, element #2=w52:string, element #3=w53:string)
      n164 = call-poly <userlib>:"gfitsio-write-key.vi"("comment"=w54, "keyname"=w56, "error in (no error)"=w60, "value"=w55, "gfits refnum"=w61) -> ("error out"=w47:errorcluster, "dup gfits refnum"=w46:T3)  [unwired: 5 in]
      n165 = call-poly <userlib>:"gfitsio-write-key.vi"("comment"=w53, "keyname"=w51, "error in (no error)"=w47, "value"=w52, "gfits refnum"=w46) -> ("error out"=w16:errorcluster, "dup gfits refnum"=w15:T3)  [unwired: 5 in]
      n166 = call <userlib>:"gfitsio-close-file.vi"("error in (no error)"=w16, "gfits refnum"=w15) -> ("error out"=w699:errorcluster)  [unwired: 8 in, 1 out]
    }
    frame Error {
    }
  }
  "error out" <- w4
  "CCDCamera out" <- w3
